vi "Tree Value FG.vi"(7 "Get Set Enum":enum16{"Get", "Set", "Clear"}(ring), 10 "NewVal":string[](array[string]), 11 "Old Val":string[](array[string])) -> (3 "Compiled Value":string[](array[string]))   [LabVIEW 2023]
uses:
  <userlib>/_OpenG.lib/array/array.llb/Filter 1D Array (String)__ogtk.vi
  <userlib>/_OpenG.lib/array/array.llb/openg_array.lvlib
panel:
  out "added elements":string[](array[string])
  out "removed elements":string[](array[string])
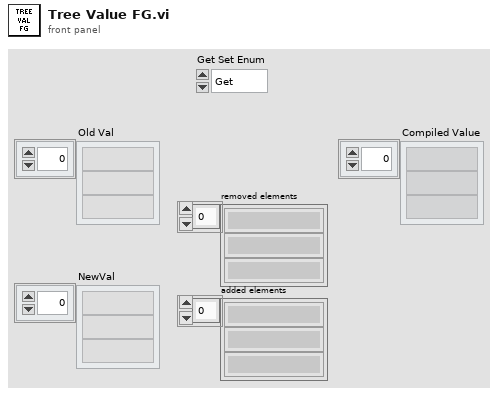
[diagram p1: front panel]
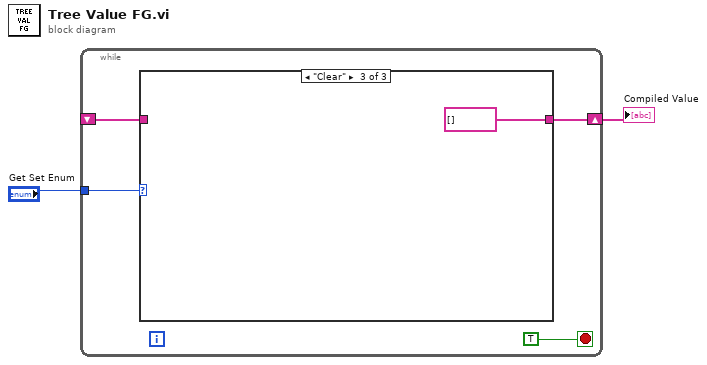
[diagram p0: block diagram]
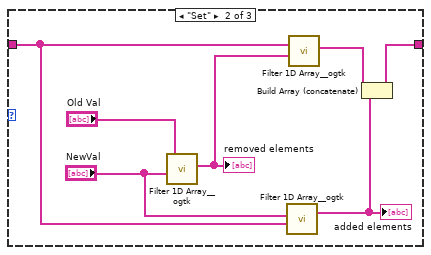
[diagram p3: hidden frame]
diagram:
  n1 = while {
    shift-right: [w4] -> w2
    shift-left: _ -> [w5]
    tunnel: "Get Set Enum" -> [w3]
    stop <- TRUE stop-if-true
    n2 = case shown="\"Clear\"" w3 {
      tunnel: w5 -> [w7 w11 _]
      tunnel: [w7 w9 string[] []] -> w4
      frame "Get", Default {
      }
      frame "Set" {
        n3 = call-poly <userlib>:"Filter 1D Array__ogtk.vi"("items to filter"="NewVal", "array"="Old Val") -> ("filtered array"=w13:string[])  [unwired: 4 in, 1 out]
        "removed elements" <- w13
        n4 = call-poly <userlib>:"Filter 1D Array__ogtk.vi"("items to filter"=w11, "array"="NewVal") -> ("filtered array"=w8:string[])  [unwired: 4 in, 1 out]
        "added elements" <- w8
        n5 = call-poly <userlib>:"Filter 1D Array__ogtk.vi"("items to filter"=w13, "array"=w11) -> ("filtered array"=w10:string[])  [unwired: 4 in, 1 out]
        n6 = Build Array (concatenate)(w10, w8) -> (w9:string[])
      }
      frame "Clear" {
      }
    }
  }
  "Compiled Value" <- w2
